vi "State_Machine.vi"(8 "error in (no error)":errorcluster caption="entrée d'erreur (pas d'erreur)", 11 "Flash_AVRDUDE en entrée":refnum<class "Flash_Commander.lvclass">) -> (0 "error out":errorcluster caption="sortie d'erreur", 2 "Json_String":string, 3 "Flash_AVRDUDE en sortie":refnum<class "Flash_Commander.lvclass">)   [LabVIEW 2020, in "Library Test.lvlib" / "Flash_Commander.lvclass"]
uses:
  Flash_Commander.lvclass
  C:/Users/ngarcin/OneDrive - Altyor/Standard TB/Class/Test/Test (Default)/Test (Default).lvclass
  Flash_Commander.lvclass/Flash_Commander.ctl
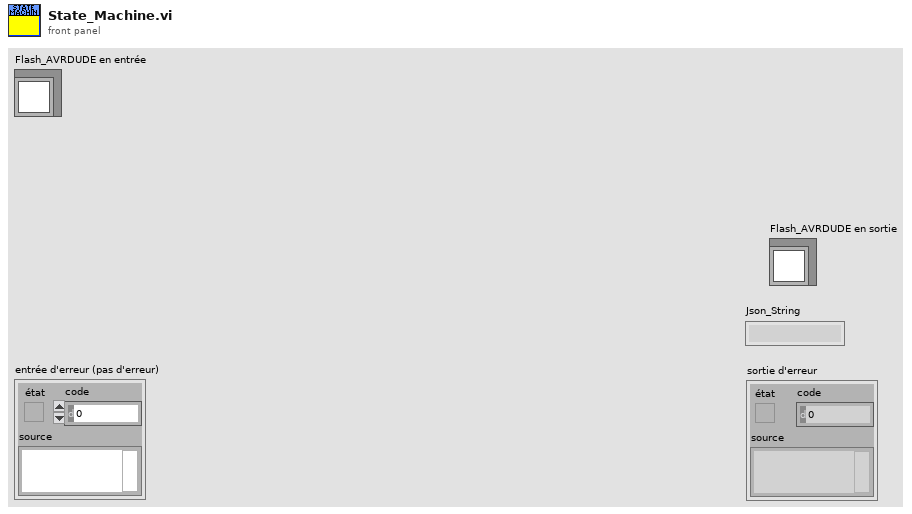
[diagram p1: front panel]
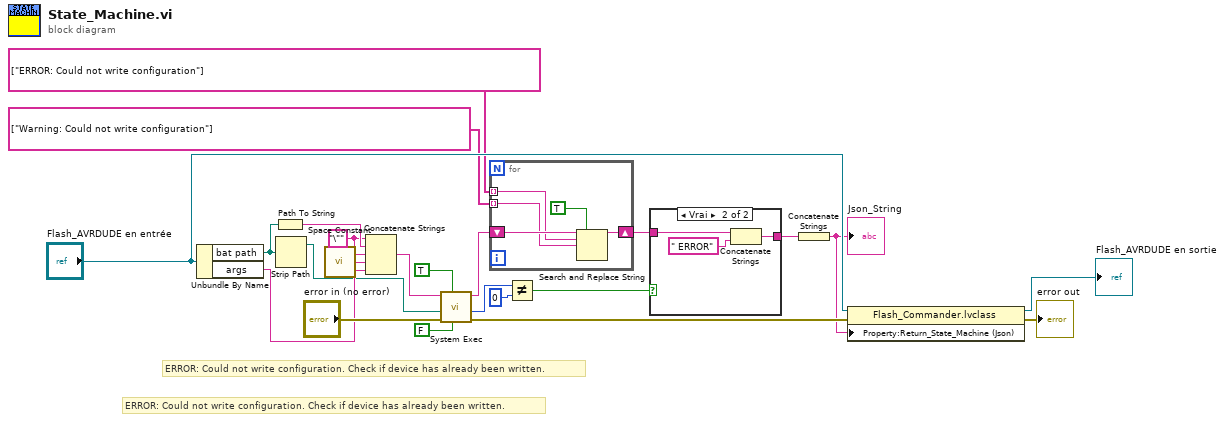
[diagram p0: block diagram]
diagram:
  w6 = "\""
  # "ERROR: Could not write configuration. Check if device has already been written."
  # "ERROR: Could not write configuration. Check if device has already been written."
  n1 = Unbundle By Name("Flash_AVRDUDE en entrée") -> ("bat path"=w11:path, "args"=w12:string)
  n2 = Path To String(path=w11) -> (string=w8:string)
  n3 = Strip Path(path=w11) -> (stripped path=w7:path)  [unwired: 1 out]
  n4 = call <vilib>:"Space Constant.vi"() -> ("String"=w13:string)
  n5 = Concatenate Strings(w6, w8, w6, w13, w12) -> (w5:string)
  n6 = call <vilib>:"System Exec.vi"("run minimized? (F)"=FALSE, "wait until completion? (T)"=TRUE, "error in (no error)"="error in (no error)", "working directory"=w7, "command line"=w5) -> ("error out"=w17:errorcluster, "return code"=w10:i32, "standard output"=w4:string)  [unwired: 3 in, 1 out]
  n7 = for {
    shift-right: [w27] -> w3
    shift-left: w4 -> [w28]
    tunnel: string[] ["ERROR: Could not write configuration"] -> [w26] mode=indexing
    tunnel: string[] ["Warning: Could not write configuration"] -> [w25] mode=indexing
    n8 = Search and Replace String(replace all?=TRUE ("tout remplacer ? (F)"), input string=w28, search string=w26, replace string=w25) -> (result string=w27:string)  [unwired: 4 in, 3 out]
  }
  n9 = Not Equal?(x=w10, y=0) -> (x != y?=w15:bool)
  n10 = case shown="Vrai" w15 {
    tunnel: w3 -> [w29 w32]
    tunnel: [w29 w30] -> w14
    frame False {
    }
    frame True {
      n11 = Concatenate Strings(w32, " ERROR" ("expression régulière")) -> (w30:string)
    }
  }
  n12 = Concatenate Strings(w14) -> (w9:string)
  "Json_String" <- w9
  n13 = property class="Flash_Commander.lvclass"(reference="Flash_AVRDUDE en entrée", error in=w17, "Property:Return_State_Machine (Json)"=w9) -> (reference out=→"Flash_AVRDUDE en sortie":refnum<class "Flash_Commander.lvclass">, error out=→"error out":errorcluster)
